vi "niFpgaXIPINGlobal.vi"() -> ()   [LabVIEW 2017]
panel:
  in  "MAXIMUM BD Node WIDTH":i16=92
  in  "MAXIMUM PATH LENGTH":i32=192
  out "CONTRACTED VIEW":picture
  out "EXCLAMATATION":picture
  in  "OVERCLOCK ID":string="ni_overclock_unique_id"
  out "LOGO":picture
  in  "CONFIG PAGE4 ID":string="XIPIN_MENU_CONFIG_PAGE4"
  in  "CONFIG PAGE3 ID":string="XIPIN_MENU_CONFIG_PAGE3"
  in  "CONFIG PAGE2 ID":string="XIPIN_MENU_CONFIG_PAGE2"
  in  "CONFIG PAGE1 ID":string="XIPIN_MENU_CONFIG_PAGE1"
  in  "CONFIG MENU ID":string="IPIN_MENU_CONFIG"
  in  "SMALL ICON MENU ID":string="XIPIN_MENU_SMALL_ICON"
  in  "BIG ICON MENU ID":string="XIPIN_MENU_BIG_ICON"
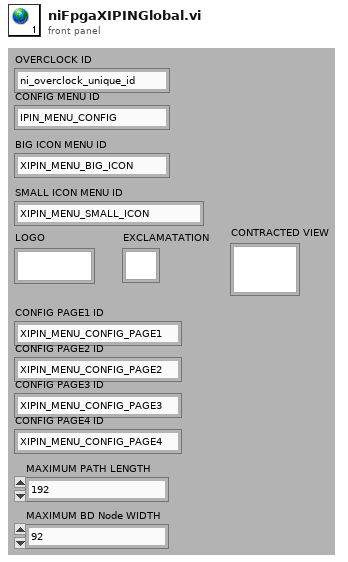
[diagram p1: front panel]
diagram:
